vi "construtor.vi"(8 "error in (no error)":errorcluster, 10 "device":refnum<class "device.lvclass">) -> (0 "error out":errorcluster, 3 "DeviceData out":refnum<class "DeviceData.lvclass">)   [LabVIEW 2009, in "DataMappers.lvlib" / "DeviceData.lvclass"]
uses:
  DeviceData.lvclass
  DatabaseHelpers/Database Objects/device/device.lvclass
  DoDeviceData/DoDeviceData.lvclass
  AoDeviceData/AoDeviceData.lvclass
  RfOutputData/RfOutputData.lvclass
  DeviceData.lvclass/DeviceData.ctl
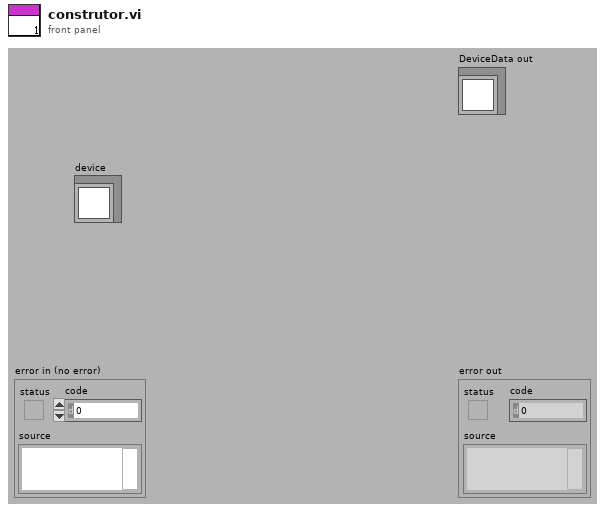
[diagram p1: front panel]
types:
  T1 = enum16{"digitalOutput", "digitalInput", "analogOutput", "analogInput", "rfOutput", "ethernetSupply"}
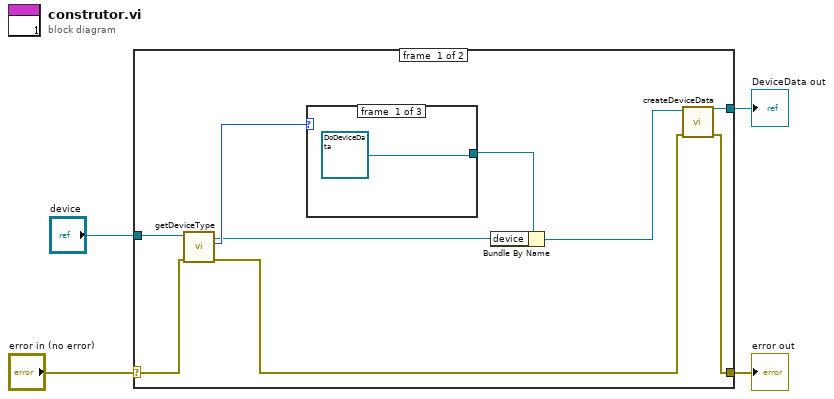
[diagram p0: block diagram]
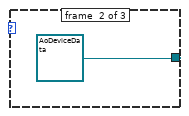
[diagram p2: hidden frame]
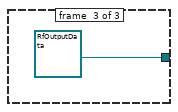
[diagram p3: hidden frame]
diagram:
  n1 = case shown="No Error" "error in (no error)" {
    selector: "error in (no error)" -> [w12 w17]
    tunnel: [w5 w17] -> w3
    tunnel: [w7 _] -> w1
    tunnel: "device" -> [w13 _]
    frame #0 {
      n2 = call-dynamic "getDeviceType.vi"("error in (no error)"=w12, "device.lvclass in"=w13) -> ("error out"=w6:errorcluster, "type"=w11:T1, "device.lvclass out"=w9:refnum<class "device.lvclass">)  [unwired: 7 in]
      n3 = case shown="\"rfOutput\"" w11 {
        tunnel: [refnum<class "DoDeviceData.lvclass"> refnum ("DataMappers.lvlib:DoDeviceData.lvclass") refnum<class "AoDeviceData.lvclass"> refnum ("DataMappers.lvlib:AoDeviceData.lvclass") refnum<class "RfOutputData.lvclass"> refnum ("DataMappers.lvlib:RfOutputData.lvclass")] -> w10
        frame #0 {
        }
        frame #1 {
        }
        frame #2 {
        }
      }
      n4 = Bundle By Name(cluster=w10, "device"=w9) -> (w8:refnum<class "DeviceData.lvclass">)
      n5 = call-dynamic "createDeviceData.vi"("error in (no error)"=w6, "DeviceData in"=w8) -> ("error out"=w5:errorcluster, "DeviceData out"=w7:refnum<class "DeviceData.lvclass">)  [unwired: 8 in]
    }
    frame #1 {
    }
  }
  "error out" <- w3
  "DeviceData out" <- w1
